vi "ULS Andor CCD.vi"(8 "error in (no error)":errorcluster, 9 "Array Data":T2, 10 "General Info":T1={"CCD Model Num"="", "Exposure time(ms)"=0.0, "Average"=1, "Boxcar"=0, "Pixel Count"=1, "Readout Mode"=enum."2D", "Spec Mode"=enum."Wavelength(nm)", "Grating Groove"=1200, "Blaze"=500, "Data BG"=enum."No BG", "Ref BG"=enum."No BG", "Data Processed"=enum."No Ref", "Process Method"=enum."Not Selected", "Real Y"=0.0, "Real X"=0.0}, 11 "IFD in":refnum<class "IFD.lvclass">) -> (0 "error out":errorcluster, 3 "IFD out":refnum<class "IFD.lvclass">)   [LabVIEW 2016, in "IFD.lvclass"]
uses:
  IFD.lvclass
  Tag/IFD_Tag.lvclass/IFD_Tag.ctl
  Tag/IFD_Tag.lvclass
  IFD.lvclass/IFD.ctl
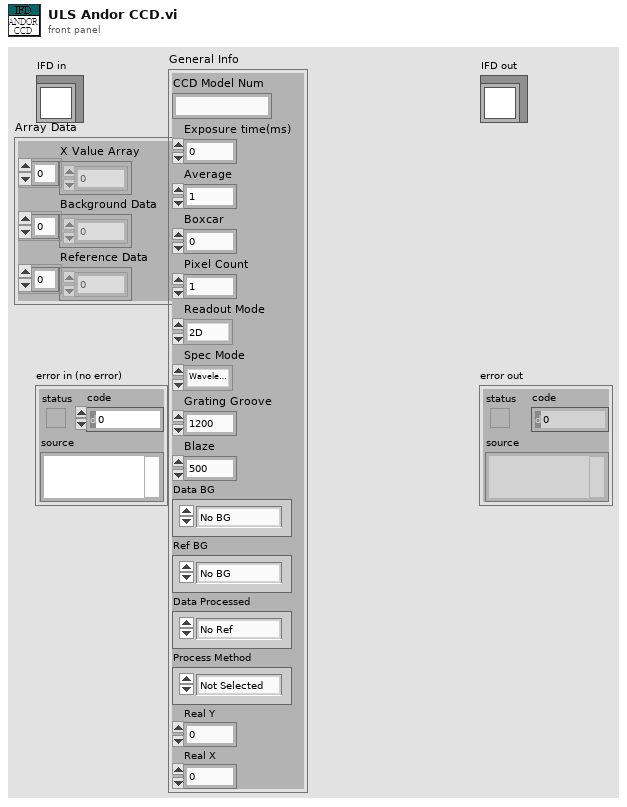
[diagram p1: front panel]
types:
  T1 = cluster{"CCD Model Num":string, "Exposure time(ms)":sgl, "Average":u8, "Boxcar":u8, "Pixel Count":u32, "Readout Mode":enum8{"FVB", "Multi Track", "Random Track", "Single Track", "2D"}, "Spec Mode":enum8{"Wavelength(nm)", "Wavenumber(/cm)"}, "Grating Groove":u16, "Blaze":u16, "Data BG":enum8{"No BG", "Not Subtracted", "Subtracted"}, "Ref BG":enum8{"No BG", "Not Subtracted", "Subtracted"}, "Data Processed":enum8{"No Ref", "Not Processed", "Processed"}, "Process Method":enum8{"Not Selected", "Absorption", "Transmission", "Subtraction"}, "Real Y":dbl, "Real X":dbl}
  T2 = cluster{"X Value Array":sgl[], "Background Data":u16[], "Reference Data":u16[]}
  T3 = enum16{"big-endian, network order", "native, host order", "little-endian"}
  T4 = enum16{"Undefined(DO NOT USE)", "U8", "ASCII", "U16", "U32", "RATIONAL", "I8", "Undefined 8 bit", "I16", "I32", "SRATIONAL", "SGL", "DBL"}
  T5 = enum8{"FVB", "Multi Track", "Random Track", "Single Track", "2D"}
  T6 = enum8{"Not Selected", "Absorption", "Transmission", "Subtraction"}
  T7 = cluster{"Data BG":enum8{"No BG", "Not Subtracted", "Subtracted"}, "Ref BG":enum8{"No BG", "Not Subtracted", "Subtracted"}, "Data Processed":enum8{"No Ref", "Not Processed", "Processed"}, "Process Method":enum8{"Not Selected", "Absorption", "Transmission", "Subtraction"}}
  T8 = cluster{"Spec Mode":enum8{"Wavelength(nm)", "Wavenumber(/cm)"}, "Average":u8, "Boxcar":u8, "Readout Mode":enum8{"FVB", "Multi Track", "Random Track", "Single Track", "2D"}}
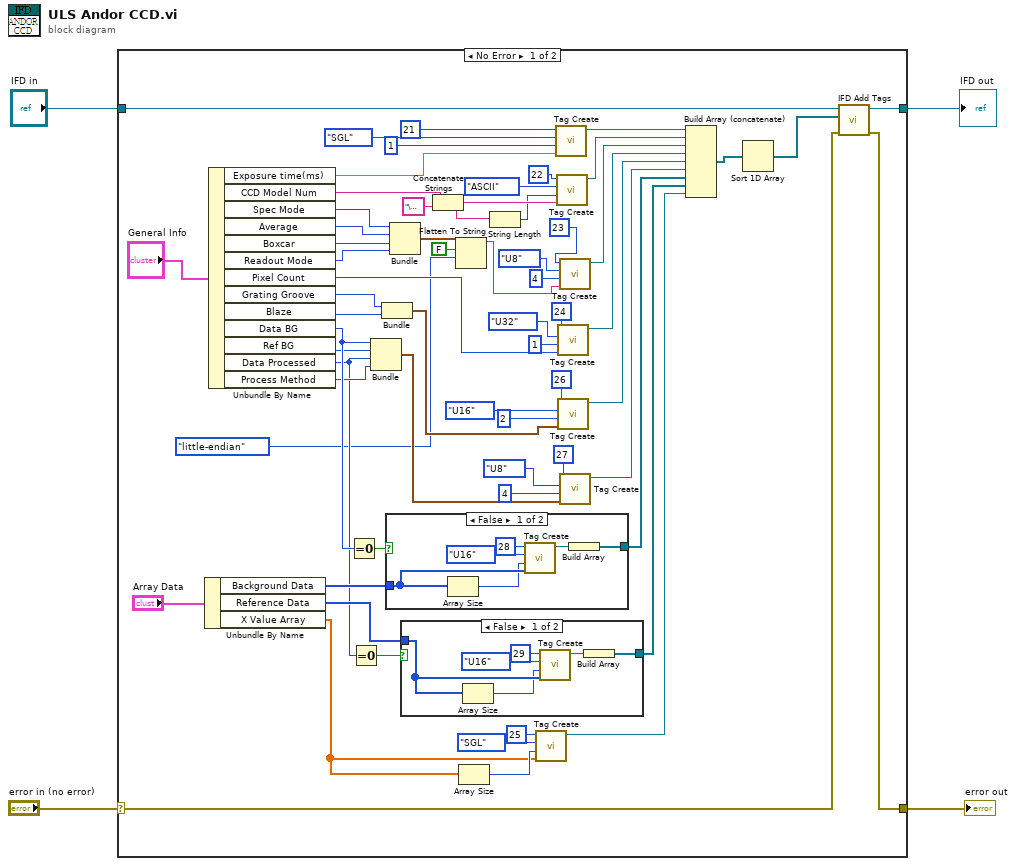
[diagram p0: block diagram]
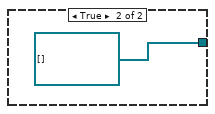
[diagram p2: hidden frame]
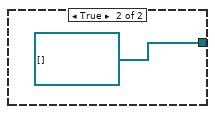
[diagram p3: hidden frame]
diagram:
  n1 = case shown="No Error" "error in (no error)" {
    selector: "error in (no error)" -> [w68 w84]
    tunnel: [w67 w84] -> w3
    tunnel: [w66 w83] -> w1
    tunnel: "IFD in" -> [w65 w83]
    frame No Error {
      n2 = Unbundle By Name("Array Data") -> ("Background Data"=w27:u16[], "Reference Data"=w24:u16[], "X Value Array"=w19:sgl[])
      n3 = Unbundle By Name("General Info") -> ("Exposure time(ms)"=w54:sgl, "CCD Model Num"=w51:string, "Spec Mode"=w8:enum8{"Wavelength(nm)", "Wavenumber(/cm)"}, "Average"=w7:u8, "Boxcar"=w6:u8, "Readout Mode"=w5:T5, "Pixel Count"=w40:u32, "Grating Groove"=w39:u16, "Blaze"=w38:u16, "Data BG"=w30:enum8{"No BG", "Not Subtracted", "Subtracted"}, "Ref BG"=w18:enum8{"No BG", "Not Subtracted", "Subtracted"}, "Data Processed"=w16:enum8{"No Ref", "Not Processed", "Processed"}, "Process Method"=w17:T6)
      n4 = Equal To 0?(x=w30) -> (x = 0?=w28:bool)
      n5 = Equal To 0?(x=w16) -> (x = 0?=w25:bool)
      n6 = Bundle("Data BG"=w30, "Ref BG"=w18, "Data Processed"=w16, "Process Method"=w17) -> (w31:T7)  [unwired: 1 in]
      n7 = Bundle("Grating Groove"=w39, "Blaze"=w38) -> (w36:cluster{"Grating Groove":u16, "Blaze":u16})  [unwired: 1 in]
      n8 = case shown="False" w28 {
        tunnel: [w80 refnum<class "IFD_Tag.lvclass">[] []] -> w29
        tunnel: w27 -> [w77 _]
        frame False {
          n9 = Array Size(array=w77) -> (size(s)=w76:i32)
          n10 = call "Tag Create.vi"("Data"=w77, "Data Count"=w76, "Data Type"=T4."U16", "Tag ID"=u16 28) -> ("IFD_Tag out"=w81:refnum<class "IFD_Tag.lvclass">)  [unwired: 7 in]
          n11 = Build Array(w81) -> (w80:refnum<class "IFD_Tag.lvclass">[])
        }
        frame True {
        }
      }
      n12 = Bundle("Spec Mode"=w8, "Average"=w7, "Boxcar"=w6, "Readout Mode"=w5) -> (w44:T8)  [unwired: 1 in]
      n13 = case shown="False" w25 {
        tunnel: [w73 refnum<class "IFD_Tag.lvclass">[] []] -> w26
        tunnel: w24 -> [w70 _]
        frame False {
          n14 = Array Size(array=w70) -> (size(s)=w69:i32)
          n15 = call "Tag Create.vi"("Data"=w70, "Data Count"=w69, "Data Type"=T4."U16", "Tag ID"=u16 29) -> ("IFD_Tag out"=w74:refnum<class "IFD_Tag.lvclass">)  [unwired: 7 in]
          n16 = Build Array(w74) -> (w73:refnum<class "IFD_Tag.lvclass">[])
        }
        frame True {
        }
      }
      n17 = Concatenate Strings(w51, "\u0000") -> (w49:string)
      n18 = Flatten To String(anything=w44, prepend array or string size? (T)=FALSE, byte order (0:big-endian, network order)=T3."little-endian") -> (data string=w13:string)  [unwired: 1 in, 2 out]
      n19 = Array Size(array=w19) -> (size(s)=w23:i32)
      n20 = String Length(string=w49) -> (length=w48:i32)
      n21 = call "Tag Create.vi"("Data"=w19, "Data Count"=w23, "Data Type"=T4."SGL", "Tag ID"=u16 25) -> ("IFD_Tag out"=w20:refnum<class "IFD_Tag.lvclass">)  [unwired: 7 in]
      n22 = call "Tag Create.vi"("Data"=w54, "Data Count"=u32 1, "Data Type"=T4."SGL", "Tag ID"=u16 21) -> ("IFD_Tag out"=w64:refnum<class "IFD_Tag.lvclass">)  [unwired: 7 in]
      n23 = call "Tag Create.vi"("Data"=w49, "Data Count"=w48, "Data Type"=T4."ASCII", "Tag ID"=u16 22) -> ("IFD_Tag out"=w59:refnum<class "IFD_Tag.lvclass">)  [unwired: 7 in]
      n24 = call "Tag Create.vi"("Data"=w40, "Data Count"=u32 1, "Data Type"=T4."U32", "Tag ID"=u16 24) -> ("IFD_Tag out"=w57:refnum<class "IFD_Tag.lvclass">)  [unwired: 7 in]
      n25 = call "Tag Create.vi"("Data"=w36, "Data Count"=u32 2, "Data Type"=T4."U16", "Tag ID"=u16 26) -> ("IFD_Tag out"=w56:refnum<class "IFD_Tag.lvclass">)  [unwired: 7 in]
      n26 = call "Tag Create.vi"("Data"=w13, "Data Count"=u32 4, "Data Type"=T4."U8", "Tag ID"=u16 23) -> ("IFD_Tag out"=w58:refnum<class "IFD_Tag.lvclass">)  [unwired: 7 in]
      n27 = call "Tag Create.vi"("Data"=w31, "Data Count"=u32 4, "Data Type"=T4."U8", "Tag ID"=u16 27) -> ("IFD_Tag out"=w55:refnum<class "IFD_Tag.lvclass">)  [unwired: 7 in]
      n28 = Build Array (concatenate)(w64, w59, w58, w57, w56, w55, w29, w26, w20) -> (w10:refnum<class "IFD_Tag.lvclass">[])
      n29 = Sort 1D Array(array=w10) -> (sorted array=w9:refnum<class "IFD_Tag.lvclass">[])
      n30 = call "IFD Add Tags.vi"("error in (no error)"=w68, "Tag(s)"=w9, "IFD in"=w65) -> ("error out"=w67:errorcluster, "IFD out"=w66:refnum<class "IFD.lvclass">)  [unwired: 7 in]
    }
    frame Error {
    }
  }
  "error out" <- w3
  "IFD out" <- w1
